vi "Select Voltage From Wavelength.vi"(8 "Voltages":dbl[][](array[numeric])=[[0.0, 0.0, 0.0], [5.0, 3.0, 4.0], [10.0, 6.0, 8.0]] min=0.0 max=360.0 step=0.1 format="%0.3f", 9 "Mode":i16, 10 "Wavelength":i16, 11 "SIM Frame":i16) -> (2 "Voltage out":dbl)   [LabVIEW 2018]
panel:
  # "0: 488\n1: 561\n2: 640"
  # "0: W-f\n1: TIRF\n2: SIM\n3: TIRF-SIM"
  # "Voltage #"
  # "Wavelength #"
  # "0: 488\n1: 561\n2: 640"
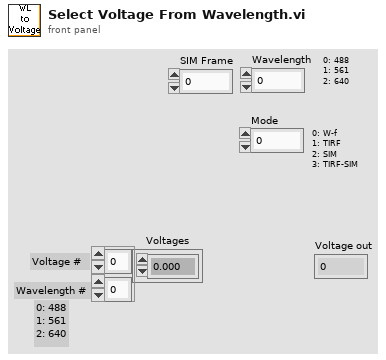
[diagram p1: front panel]
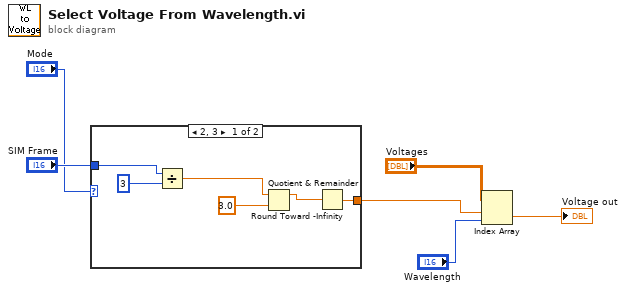
[diagram p0: block diagram]
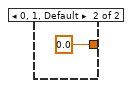
[diagram p2: hidden frame]
diagram:
  n1 = case shown="2, 3" "Mode" {
    tunnel: "SIM Frame" -> [w12 _]
    tunnel: [w7 0.0] -> w4
    frame 2, 3 {
      n2 = Divide(x=w12, y=i16 3) -> (x/y=w10:dbl)
      n3 = Quotient & Remainder(x=w10, y=3.0) -> (x-y*floor(x/y)=w8:dbl)  [unwired: 1 out]
      n4 = Round Toward -Infinity(1:w8) -> (0:w7:dbl)
    }
    frame 0, 1, Default {
    }
  }
  n5 = Index Array(array="Voltages", index (row)=w4, index (col)="Wavelength") -> (element=→"Voltage out":dbl)
